vi "SolveBestPath.vi"(8 "error in (no error)":errorcluster, 11 "RouteTree in":refnum<class "RouteTree.lvclass">) -> (0 "error out":errorcluster, 1 "found":bool, 2 "Path":T1[](array[typedef]), 3 "RouteTree out":refnum<class "RouteTree.lvclass">)   [LabVIEW 2013, in "RouteTree.lvclass"]
uses:
  RouteTree.lvclass
  Waypoint/point.ctl
  Tree/SearchMethod.ctl
  Waypoint/Waypoint.lvclass
  Tree/Tree.lvclass
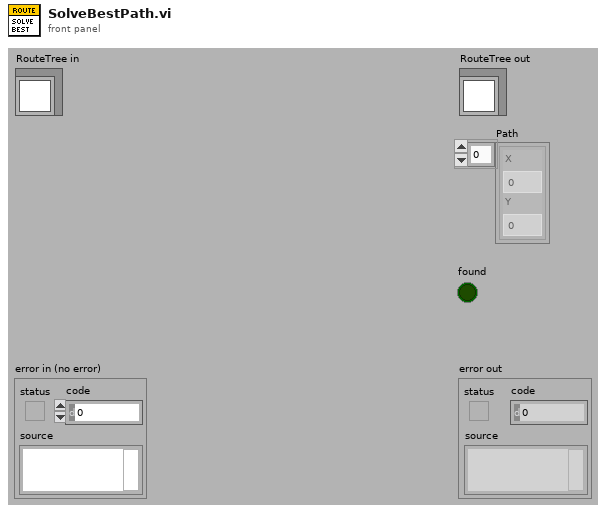
[diagram p1: front panel]
types:
  T1 = typedef "Waypoint.lvclass/point.ctl" = cluster{"X":dbl, "Y":dbl}
  T2 = typedef "Tree.lvclass/SearchMethod.ctl" = enum16{"Breadth (First)", "Depth (First)", "Best First", "Breadth (Exhaustive)", "Depth (Exhaustive)"}
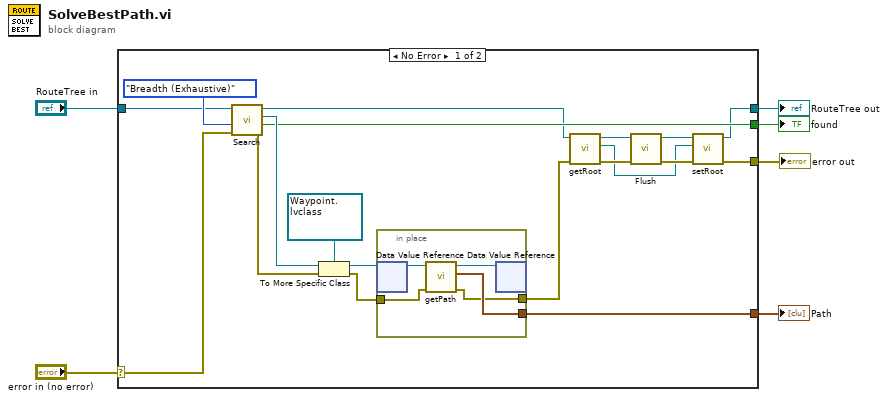
[diagram p0: block diagram]
diagram:
  n1 = case shown="No Error" "error in (no error)" {
    selector: "error in (no error)" -> [w18 w32]
    tunnel: [w8 w32] -> w5
    tunnel: [w10 w31] -> w3
    tunnel: "RouteTree in" -> [w20 w31]
    tunnel: [w19 _] -> w2
    tunnel: [w17 _] -> w1
    frame No Error {
      n2 = call "Search.vi"("error in (no error)"=w18, "SearchMethod"=SearchMethod."Breadth (Exhaustive)", "Tree in"=w20) -> ("error out"=w21:errorcluster, "found"=w19:bool, "Node"=w23:refnum<data-value>, "Tree out"=w16:refnum<class "RouteTree.lvclass">)  [unwired: 5 in]
      n3 = To More Specific Class(target class=refnum<data-value> refnum ("data value reference"), reference=w23, error in=w21) -> (specific class reference=w24:refnum<data-value>, error out=w13:errorcluster)
      n4 = in-place {
        in-place-border: [w28] -> w17
        in-place-border: w13 -> [w27]
        in-place-border: [w26] -> w12
        n5 = in-place-dvr #1(w24) -> (w30:refnum<class "Waypoint.lvclass">)  [unwired: 1 out]
        n6 = call "getPath.vi"("error in (no error)"=w27, "Waypoint in"=w30) -> ("error out"=w26:errorcluster, "Path"=w28:T1[], "Waypoint out"=w29:refnum<class "Waypoint.lvclass">)  [unwired: 7 in]
        n7 = in-place-dvr #1(w29) -> ()  [unwired: 2 out]
      }
      n8 = call "getRoot.vi"("error in (no error)"=w12, "Tree in"=w16) -> ("error out"=w14:errorcluster, "Root"=w7:refnum<data-value>, "Tree out"=w15:refnum<class "RouteTree.lvclass">)  [unwired: 7 in]
      n9 = call "Flush.vi"("error in (no error)"=w14, "Tree in"=w15) -> ("error out"=w9:errorcluster, "Tree out"=w11:refnum<class "RouteTree.lvclass">)  [unwired: 7 in, 1 out]
      n10 = call "setRoot.vi"("error in (no error)"=w9, "Root"=w7, "Tree in"=w11) -> ("error out"=w8:errorcluster, "Tree out"=w10:refnum<class "RouteTree.lvclass">)  [unwired: 7 in]
    }
    frame Error {
    }
  }
  "error out" <- w5
  "RouteTree out" <- w3
  "found" <- w2
  "Path" <- w1
